vi "test_libssh2_sftp_open_ex (create).vi"() -> ()   [LabVIEW 2013, in "libssh2_integration_tests.lvlib"]
uses:
  libssh2_integration_tests.lvlib
  <vilib>/addons/_JKI Toolkits/Caraya/classes/Test/Test.lvclass
  support/support.lvlib
  <vilib>/addons/_JKI Toolkits/Caraya/classes/Assert/Assert.lvclass
  libssh2/libssh2.lvlib
panel:
  out "error out":errorcluster
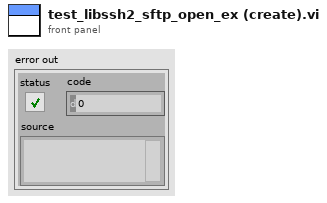
[diagram p1: front panel]
types:
  T1 = typedef "libssh2.lvlib/Session Refnum.ctl" = refnum<k1>
  T2 = typedef "libssh2.lvlib/SFTP Refnum.ctl" = refnum<k1>
  T3 = typedef "libssh2.lvlib/SFTP Handle Refnum.ctl" = refnum<k1>
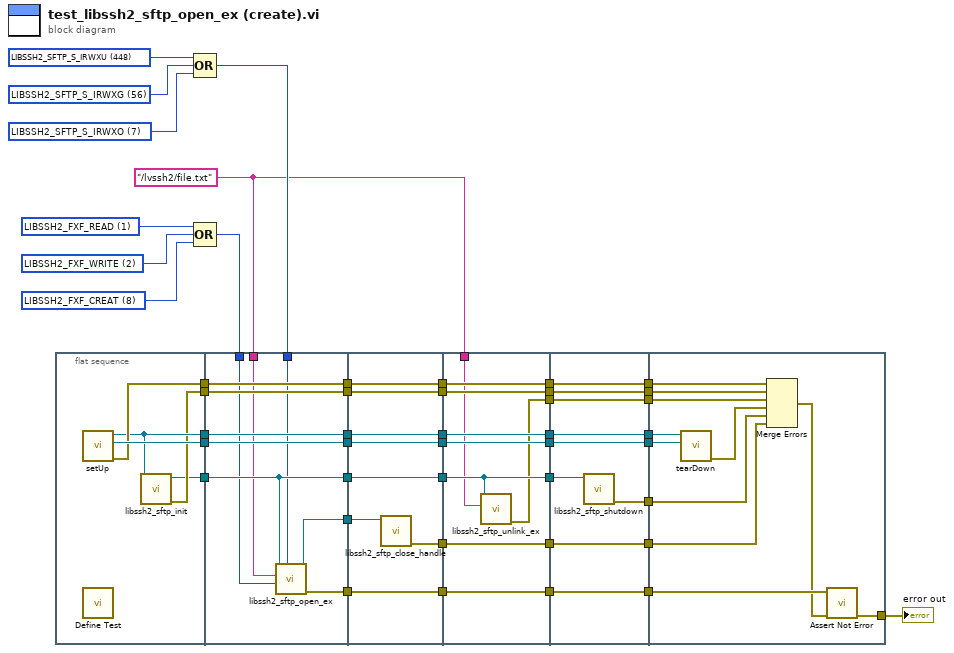
[diagram p0: block diagram]
diagram:
  w34 = u32 2 items=["LIBSSH2_FXF_READ"=1, "LIBSSH2_FXF_WRITE"=2, "LIBSSH2_FXF_APPEND"=4, "LIBSSH2_FXF_CREAT"=8, "LIBSSH2_FXF_TRUNC"=16, "LIBSSH2_FXF_EXCL"=32] ("flags")
  w35 = u32 1 items=["LIBSSH2_FXF_READ"=1, "LIBSSH2_FXF_WRITE"=2, "LIBSSH2_FXF_APPEND"=4, "LIBSSH2_FXF_CREAT"=8, "LIBSSH2_FXF_TRUNC"=16, "LIBSSH2_FXF_EXCL"=32] ("flags")
  w33 = u32 8 items=["LIBSSH2_FXF_READ"=1, "LIBSSH2_FXF_WRITE"=2, "LIBSSH2_FXF_APPEND"=4, "LIBSSH2_FXF_CREAT"=8, "LIBSSH2_FXF_TRUNC"=16, "LIBSSH2_FXF_EXCL"=32] ("flags")
  w3 = "/lvssh2/file.txt" ("filename")
  w37 = 7 items=["LIBSSH2_SFTP_S_IRWXU"=448, "LIBSSH2_SFTP_S_IRUSR"=256, "LIBSSH2_SFTP_S_IWUSR"=128, "LIBSSH2_SFTP_S_IXUSR"=64, "LIBSSH2_SFTP_S_IRWXG"=56, "LIBSSH2_SFTP_S_IRGRP"=32, "LIBSSH2_SFTP_S_IWGRP"=16, "LIBSSH2_SFTP_S_IXGRP"=8, "LIBSSH2_SFTP_S_IRWXO"=7, "LIBSSH2_SFTP_S_IROTH"=4, "LIBSSH2_SFTP_S_IWOTH"=2, "LIBSSH2_SFTP_S_IXOTH"=1] ("mode")
  w38 = 56 items=["LIBSSH2_SFTP_S_IRWXU"=448, "LIBSSH2_SFTP_S_IRUSR"=256, "LIBSSH2_SFTP_S_IWUSR"=128, "LIBSSH2_SFTP_S_IXUSR"=64, "LIBSSH2_SFTP_S_IRWXG"=56, "LIBSSH2_SFTP_S_IRGRP"=32, "LIBSSH2_SFTP_S_IWGRP"=16, "LIBSSH2_SFTP_S_IXGRP"=8, "LIBSSH2_SFTP_S_IRWXO"=7, "LIBSSH2_SFTP_S_IROTH"=4, "LIBSSH2_SFTP_S_IWOTH"=2, "LIBSSH2_SFTP_S_IXOTH"=1] ("mode")
  w39 = 448 items=["LIBSSH2_SFTP_S_IRWXU"=448, "LIBSSH2_SFTP_S_IRUSR"=256, "LIBSSH2_SFTP_S_IWUSR"=128, "LIBSSH2_SFTP_S_IXUSR"=64, "LIBSSH2_SFTP_S_IRWXG"=56, "LIBSSH2_SFTP_S_IRGRP"=32, "LIBSSH2_SFTP_S_IWGRP"=16, "LIBSSH2_SFTP_S_IXGRP"=8, "LIBSSH2_SFTP_S_IRWXO"=7, "LIBSSH2_SFTP_S_IROTH"=4, "LIBSSH2_SFTP_S_IWOTH"=2, "LIBSSH2_SFTP_S_IXOTH"=1] ("mode")
  n1 = flat-sequence {
    tunnel: [w48] -> w45
    tunnel: [w50] -> w44
    tunnel: [w49] -> w43
    tunnel: [w47] -> w41
    tunnel: [w46] -> w40
    tunnel: w45 -> [w60]
    tunnel: w44 -> [w59]
    tunnel: [w60] -> w24
    tunnel: [w59] -> w23
    tunnel: [w55] -> w22
    tunnel: [w56] -> w21
    tunnel: [w58] -> w20
    tunnel: w43 -> [w58]
    tunnel: w41 -> [w57]
    tunnel: [w57] -> w19
    tunnel: w40 -> [w55]
    tunnel: w36 -> [w54]
    tunnel: w3 -> [w53]
    tunnel: w32 -> [w52]
    tunnel: [w51] -> w18
    tunnel: w24 -> [w68]
    tunnel: [w68] -> w17
    tunnel: w23 -> [w67]
    tunnel: [w67] -> w15
    tunnel: w22 -> [w66]
    tunnel: [w66] -> w13
    tunnel: w21 -> [w65]
    tunnel: [w65] -> w11
    tunnel: w20 -> [w64]
    tunnel: [w64] -> w9
    tunnel: w19 -> [w63]
    tunnel: [w63] -> w7
    tunnel: w18 -> [w62]
    tunnel: [w61] -> w5
    tunnel: w17 -> [w77]
    tunnel: [w77] -> w16
    tunnel: w15 -> [w76]
    tunnel: [w76] -> w14
    tunnel: w13 -> [w71]
    tunnel: [w71] -> w12
    tunnel: w11 -> [w75]
    tunnel: [w75] -> w10
    tunnel: w9 -> [w74]
    tunnel: [w74] -> w8
    tunnel: w7 -> [w73]
    tunnel: [w73] -> w6
    tunnel: w5 -> [w72]
    tunnel: [w72] -> w4
    tunnel: w3 -> [w70]
    tunnel: [w69] -> w2
    tunnel: w16 -> [w86]
    tunnel: [w86] -> w31
    tunnel: w14 -> [w85]
    tunnel: [w85] -> w30
    tunnel: w12 -> [w81]
    tunnel: w10 -> [w84]
    tunnel: [w84] -> w29
    tunnel: w8 -> [w83]
    tunnel: [w83] -> w28
    tunnel: w6 -> [w82]
    tunnel: [w82] -> w27
    tunnel: [w80] -> w26
    tunnel: [w79] -> w25
    tunnel: w4 -> [w79]
    tunnel: w2 -> [w78]
    tunnel: [w78] -> w1
    tunnel: w31 -> [w97]
    tunnel: w30 -> [w96]
    tunnel: w29 -> [w95]
    tunnel: w28 -> [w94]
    tunnel: [w91] -> w42
    tunnel: w27 -> [w90]
    tunnel: w26 -> [w89]
    tunnel: w25 -> [w88]
    tunnel: w1 -> [w87]
    frame #0 {
      n2 = call "setUp.vi"() -> ("error out"=w49:errorcluster, "connection ID"=w50:refnum<k5>, "session"=w48:T1)  [unwired: 9 in]
      n3 = call <vilib>:"Define Test.vi"() -> ()  [unwired: 10 in, 2 out]
      n4 = call "libssh2_sftp_init.vi"("session"=w48) -> ("error out"=w47:errorcluster, "sftp"=w46:T2)  [unwired: 9 in]
    }
    frame #1 {
      n5 = call "libssh2_sftp_open_ex.vi"("mode"=w54, "flags"=w52, "filename"=w53, "sftp"=w55) -> ("error out"=w56:errorcluster, "sftp handle"=w51:T3)  [unwired: 6 in]
    }
    frame #2 {
      n6 = call "libssh2_sftp_close_handle.vi"("sftp handle"=w62) -> ("error out"=w61:errorcluster)  [unwired: 10 in]
    }
    frame #3 {
      n7 = call "libssh2_sftp_unlink_ex.vi"("file"=w70, "sftp"=w71) -> ("error out"=w69:errorcluster)  [unwired: 9 in]
    }
    frame #4 {
      n8 = call "libssh2_sftp_shutdown.vi"("sftp"=w81) -> ("error out"=w80:errorcluster)  [unwired: 10 in]
    }
    frame #5 {
      n9 = call "tearDown.vi"("connection ID"=w96, "session"=w97) -> ("error out"=w93:errorcluster)  [unwired: 9 in]
      n10 = Merge Errors(w94, w90, w87, w93, w89, w88) -> (w92:errorcluster)
      n11 = call <vilib>:"Assert Not Error.vi"("error in (no error)"=w92, "Not Error?"=w95) -> ("error out"=w91:errorcluster)  [unwired: 8 in, 1 out]
    }
  }
  n12 = Compound Arithmetic op=OR(w39, w38, w37) -> (w36:i32)
  n13 = Compound Arithmetic op=OR(w35, w34, w33) -> (w32:u32)
  "error out" <- w42
